vi "Messenger.vi"() -> ()   [LabVIEW 2019]
uses:
  #cluster_ApplicationData.ctl
panel:
  in  "My Port":u16=60056
  in  "Friend Port":u16=60055
  out "Connected?":bool
  in  "Friend IP Address":string="10.8.3.120"
  out "Chat":string[](array[string])
  in  "Message":string
  in  "Send":bool
  in  "Stop":bool
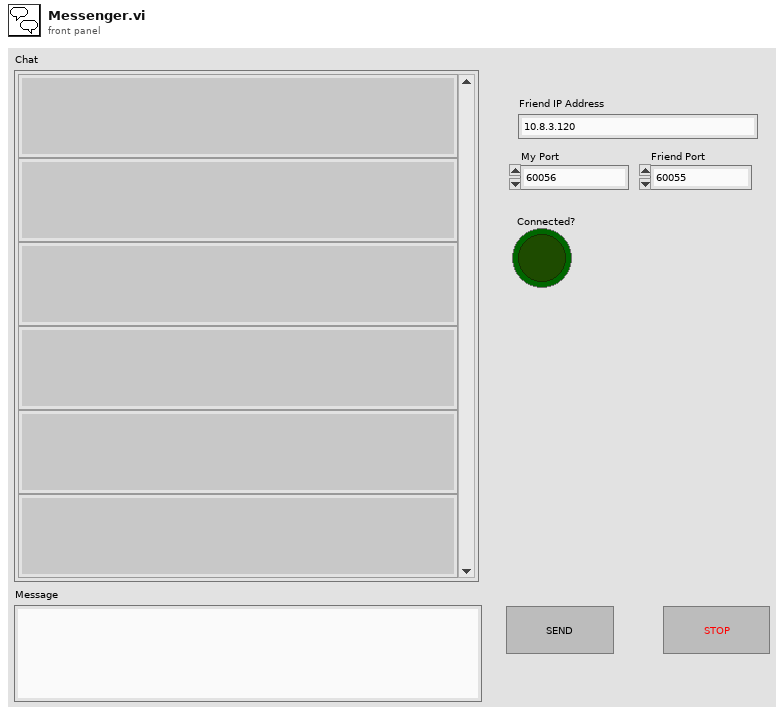
[diagram p1: front panel]
types:
  T1 = typedef "#cluster_ApplicationData.ctl" = cluster{"Connected?":bool, "Chat":string[], "connection ID":refnum<k5>}
  T2 = enum16{"Standard", "Buffered", "CRLF", "Immediate"}
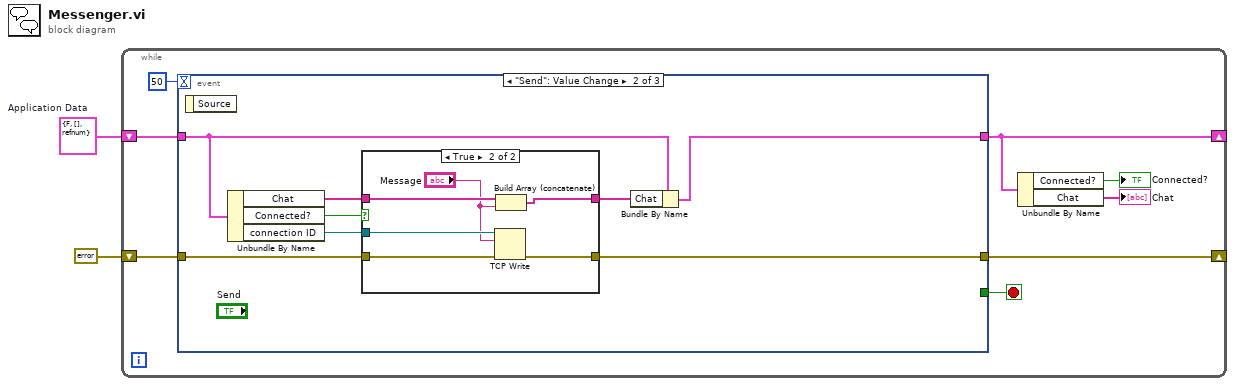
[diagram p0: block diagram]
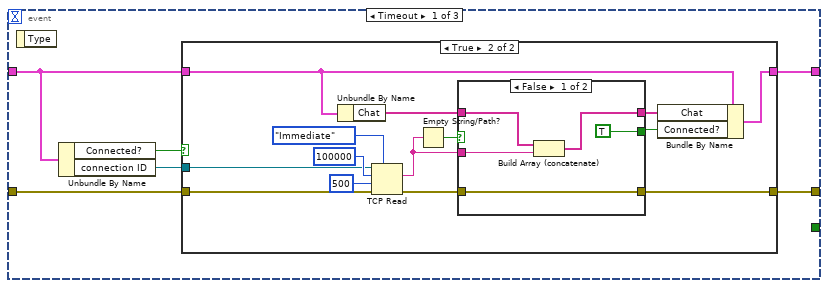
[diagram p2: hidden frame]
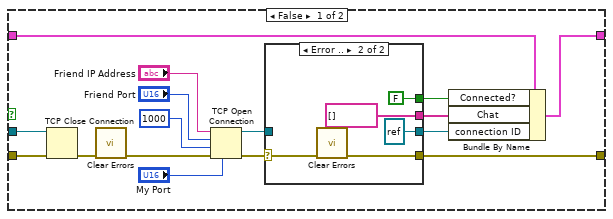
[diagram p3: hidden frame]
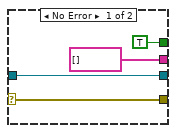
[diagram p4: hidden frame]
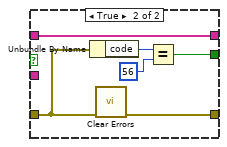
[diagram p5: hidden frame]
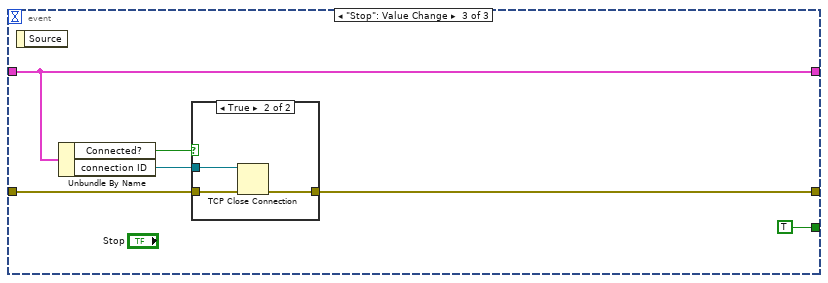
[diagram p7: hidden frame]
diagram:
  w1 = T1 {"Connected?"=FALSE, "Chat"=[], "connection ID"=refnum}  # Application Data
  n1 = while {
    shift-right: [w9] -> _
    shift-left: errorcluster {"status"=FALSE, "code"=0, "source"=""} ("error out") -> [w8]
    shift-right: [w6] -> _
    shift-left: w1 -> [w7]
    stop <- w5 stop-if-true
    n2 = event shown="[1] \"Send\": Value Change" {
      selector: _ -> [_ _ _]
      dyn-events: _ -> [_ _ _]
      timeout: 50 -> [_ _ _]
      tunnel: [_ _ TRUE ("stop")] -> w5
      tunnel: [w15 w73 w86] -> w9
      tunnel: w8 -> [w16 w74 w87]
      tunnel: w7 -> [w14 w69 w83]
      tunnel: [w12 w67 w83] -> w6
      event Timeout {
        n3 = event-data() -> ()  [unwired: 1 in, 1 out]
        n4 = Unbundle By Name(w14) -> ("Connected?"=w13:bool, "connection ID"=w11:refnum<k5>)
        n5 = case shown="True" w13 {
          tunnel: w16 -> [w20 w55]
          tunnel: [w30 w53] -> w15
          tunnel: w14 -> [w25 w46]
          tunnel: [w21 w43] -> w12
          tunnel: w11 -> [w19 w42]
          frame False {
            n6 = TCP Close Connection(connection ID=w19, error in (no error)=w20) -> (error out=w18:errorcluster)  [unwired: 1 in, 1 out]
            n7 = call <vilib>:"Clear Errors.vi"("error in (no error)"=w18) -> ("error out"=w17:errorcluster)  [unwired: 5 in, 1 out]
            n8 = TCP Open Connection(address="Friend IP Address", remote port or service name="Friend Port", timeout ms (60000)=1000, local port="My Port", error in (no error)=w17) -> (connection ID=w29:refnum<k5>, error out=w31:errorcluster)
            n9 = case shown="Error .." w31 {
              selector: w31 -> [w34 w41]
              tunnel: [w34 w40] -> w30
              tunnel: w29 -> [w36 _]
              tunnel: [w36 refnum<k5> refnum ("connection ID")] -> w22
              tunnel: [TRUE ("Connected?") FALSE ("Connected?")] -> w24
              tunnel: [string[] [] string[] []] -> w23
              frame No Error {
              }
              frame Error {
                n10 = call <vilib>:"Clear Errors.vi"("error in (no error)"=w41) -> ("error out"=w40:errorcluster)  [unwired: 5 in, 1 out]
              }
            }
            n11 = Bundle By Name(cluster=w25, "Connected?"=w24, "Chat"=w23, "connection ID"=w22) -> (w21:T1)
          }
          frame True {
            n12 = Unbundle By Name(w46) -> ("Chat"=w45:string[])
            n13 = TCP Read(connection ID=w42, bytes to read=100000, error in (no error)=w55, 7:T2."Immediate" ("mode (standard)"), 9:500 ("timeout ms (25000)")) -> (data out=w52:string, error out=w50:errorcluster)  [unwired: 1 out]
            n14 = Empty String/Path?(string/path=w52) -> (empty?=w51:bool)
            n15 = case shown="False" w51 {
              tunnel: w52 -> [w60 _]
              tunnel: [w57 w66] -> w53
              tunnel: [TRUE w61] -> w47
              tunnel: w50 -> [w57 w64]
              tunnel: w45 -> [w58 w65]
              tunnel: [w56 w65] -> w44
              frame False {
                n16 = Build Array (concatenate)(w58, w60) -> (w56:string[])
              }
              frame True {
                n17 = Unbundle By Name(w64) -> ("code"=w63:i32)
                n18 = call <vilib>:"Clear Errors.vi"("error in (no error)"=w64) -> ("error out"=w66:errorcluster)  [unwired: 5 in, 1 out]
                n19 = Equal?(x=w63, y=56) -> (x = y?=w61:bool)
              }
            }
            n20 = Bundle By Name(cluster=w46, "Chat"=w44, "Connected?"=w47) -> (w43:T1)
          }
        }
      }
      event "Send": Value Change {
        n21 = event-data() -> ()  [unwired: 1 in, 1 out]
        n22 = Unbundle By Name(w69) -> ("Chat"=w71:string[], "Connected?"=w72:bool, "connection ID"=w70:refnum<k5>)
        n23 = case shown="True" w72 {
          tunnel: w74 -> [w76 w82]
          tunnel: w70 -> [_ w81]
          tunnel: [w76 w78] -> w73
          tunnel: w71 -> [w75 w80]
          tunnel: [w75 w77] -> w68
          frame False {
          }
          frame True {
            n24 = TCP Write(connection ID=w81, data in="Message", error in (no error)=w82) -> (error out=w78:errorcluster)  [unwired: 1 in, 2 out]
            n25 = Build Array (concatenate)(w80, "Message") -> (w77:string[])
          }
        }
        n26 = Bundle By Name(cluster=w69, "Chat"=w68) -> (w67:T1)
      }
      event "Stop": Value Change {
        n27 = event-data() -> ()  [unwired: 1 in, 1 out]
        n28 = Unbundle By Name(w83) -> ("Connected?"=w85:bool, "connection ID"=w84:refnum<k5>)
        n29 = case shown="True" w85 {
          tunnel: w87 -> [w89 w92]
          tunnel: w84 -> [_ w91]
          tunnel: [w89 w90] -> w86
          frame False {
          }
          frame True {
            n30 = TCP Close Connection(connection ID=w91, error in (no error)=w92) -> (error out=w90:errorcluster)  [unwired: 1 in, 1 out]
          }
        }
      }
    }
    n31 = Unbundle By Name(w6) -> ("Connected?"=→"Connected?":bool, "Chat"=→"Chat":string[])
  }
